vi "Fix gRPC Register Dependencies.vi"(8 "error in":errorcluster, 9 "Proto Names":T1, 10 "Project Path":path, 11 "VI Refnum":refnum<vi>) -> (0 "error out":errorcluster)   [LabVIEW 2021, in "Plugin Generator.lvlib"]
uses:
  Plugin Generator.lvlib
  Typedef/Proto Names.ctl
  <vilib>/Utility/traverseref.llb/TRef TravTarget.ctl
  <vilib>/Utility/traverseref.llb/VI Scripting - Traverse.lvlib
  <vilib>/CIF Foundation/CIF LabVIEW Scripting/LV Scripting/LV Scripting Utilities.lvlib
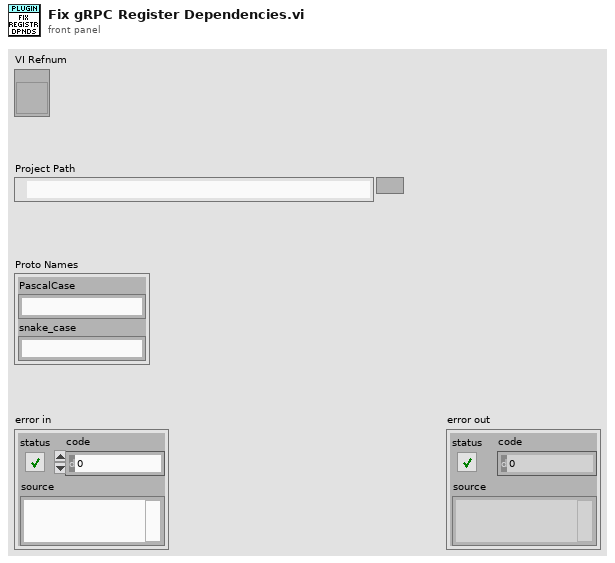
[diagram p1: front panel]
types:
  T1 = typedef "Plugin Generator.lvlib/Proto Names.ctl" = cluster{"PascalCase":string, "snake_case":string}
  T2 = typedef "TRef TravTarget.ctl" = enum16{"FP", "BD", "Other"}
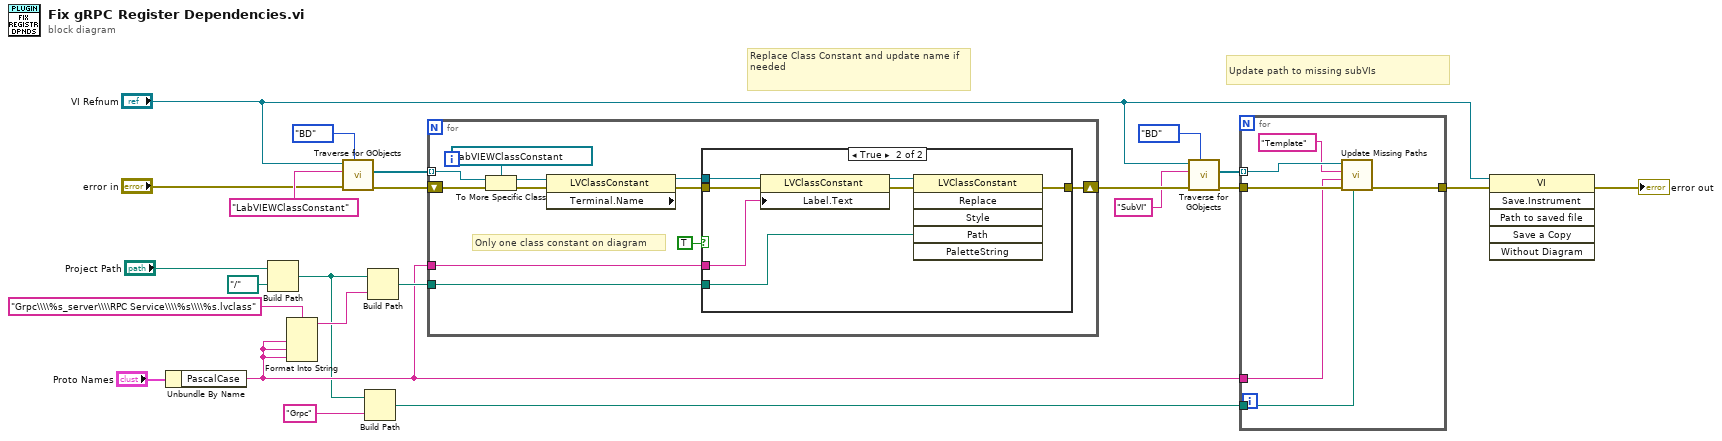
[diagram p0: block diagram]
diagram:
  # "Update path to missing subVIs"
  # "Replace Class Constant and update name if needed"
  n1 = Unbundle By Name("Proto Names") -> ("PascalCase"=w9:string)
  n2 = Build Path(base path="Project Path", name or relative path=path "../..") -> (appended path=w7:path)
  n3 = Format Into String(format string="Grpc\\\\%s_server\\\\RPC Service\\\\%s\\\\%s.lvclass" ("Class Name"), w9, w9, w9) -> (resulting string=w19:string)  [unwired: 2 in, 1 out]
  n4 = call <vilib>:"Traverse for GObjects.vi"("Traverse Target"=TRef_TravTarget."BD", "error in (no error)"="error in", "Class Name"="LabVIEWClassConstant", "VI Refnum"="VI Refnum") -> ("error out"=w14:errorcluster, "References"=w22:refnum<vi>[])  [unwired: 4 in, 2 out]
  n5 = Build Path(base path=w7, name or relative path="Grpc" ("Class Name")) -> (appended path=w6:path)
  n6 = Build Path(base path=w7, name or relative path=w19) -> (appended path=w12:path)
  n7 = for {
    tunnel: w22 -> [w34] mode=indexing
    tunnel: w9 -> [w25]
    shift-right: [w29] -> w13
    shift-left: w14 -> [w27]
    tunnel: w12 -> [w26]
    # "Only one class constant on diagram"
    n8 = To More Specific Class(target class=refnum<vi> refnum ("x"), reference=w34, error in=w27) -> (specific class reference=w28:refnum<vi>, error out=w32:errorcluster)
    n9 = property class="LVClassConstant" props=["Terminal", "Name"](reference=w28, error in=w32) -> (reference out=w30:refnum<vi>, error out=w31:errorcluster)  [unwired: 1 out]
    n10 = case shown="True" TRUE {
      tunnel: w31 -> [w35 w39]
      tunnel: w30 -> [_ w42]
      tunnel: [w35 w38] -> w29
      tunnel: w25 -> [_ w37]
      tunnel: w26 -> [_ w36]
      frame False {
      }
      frame True {
        n11 = property class="LVClassConstant"(reference=w42, error in=w39, "Label.Text"=w37) -> (reference out=w41:refnum<vi>, error out=w40:errorcluster)
        n12 = invoke class="LVClassConstant" method="Replace"(reference=w41, error in=w40, "Path"=w36) -> (error out=w38:errorcluster)  [unwired: 3 in, 5 out]
      }
    }
  }
  n13 = call <vilib>:"Traverse for GObjects.vi"("Traverse Target"=TRef_TravTarget."BD", "error in (no error)"=w13, "Class Name"="SubVI", "VI Refnum"="VI Refnum") -> ("error out"=w2:errorcluster, "References"=w3:refnum<vi>[])  [unwired: 4 in, 2 out]
  n14 = for {
    tunnel: w3 -> [w47] mode=indexing
    tunnel: w9 -> [w46]
    tunnel: w2 -> [w48]
    tunnel: [w45] -> w15
    tunnel: w6 -> [w44]
    n15 = call <vilib>:"Update Missing Paths.vi"("Search Path"=w44, "error in (no error)"=w48, "New Subname"=w46, "Subname to Replace"="Template" ("search string"), "GObject in"=w47) -> ("error out"=w45:errorcluster)  [unwired: 6 in]
  }
  n16 = invoke class="VI" method="Save.Instrument"(reference="VI Refnum", error in=w15) -> (error out=→"error out":errorcluster)  [unwired: 4 in, 5 out]
